vi "mainlockin2.vi"() -> ()   [LabVIEW 2021]
panel:
  out "outputdc 2":dbl[](array[numeric]) format="%.2f"
  in  "GPIB address dc meter 2":string
  out "dup directory path":path
  in  "GPIB address dc meter":string
  in  "GPIB  address  lockin":string
  in  "GPIB address magnet":string
  in  "GPIB address Temp controller":string
  in  "Wait (minute)":sgl
  in  "No of Temp Steps":i16
  in  "folder name to save files":string
  out "outputtemp":dbl[](array[numeric]) format="%.2f"
  out "outputdc":dbl[](array[numeric]) format="%.2f"
  out "outputlockin 2":dbl[](array[numeric]) format="%.2f"
  out "outputlockin 1":dbl[](array[numeric]) format="%.2f"
  out "field":dbl[](array[numeric]) format="%.2f"
  out "Current Temp":dbl format="%.3f"
  in  "Increasing \nTemp step":bool=TRUE
  in  "Temperature\nInterval":dbl format="%.3f"
  in  "Initial Temp C":dbl format="%.3f"
  # "Help:\n1. write the folder name to save the files.The file name will \nbe the temperature in the given folder.\n2.Write the GPIB address of all the instruments before running\nthe program.\n3. Give the initial temperature and the temperature interval \nand the total number of steps.\n4.Check whether you want to increase the temperature or\ndecrease.\n5.Write the time to be waited to let the tempetature controller\nequilibrate.\n6.Once the speps 1 through 5 is done run the experiment."
  # "Decreasing\nTemp Step"
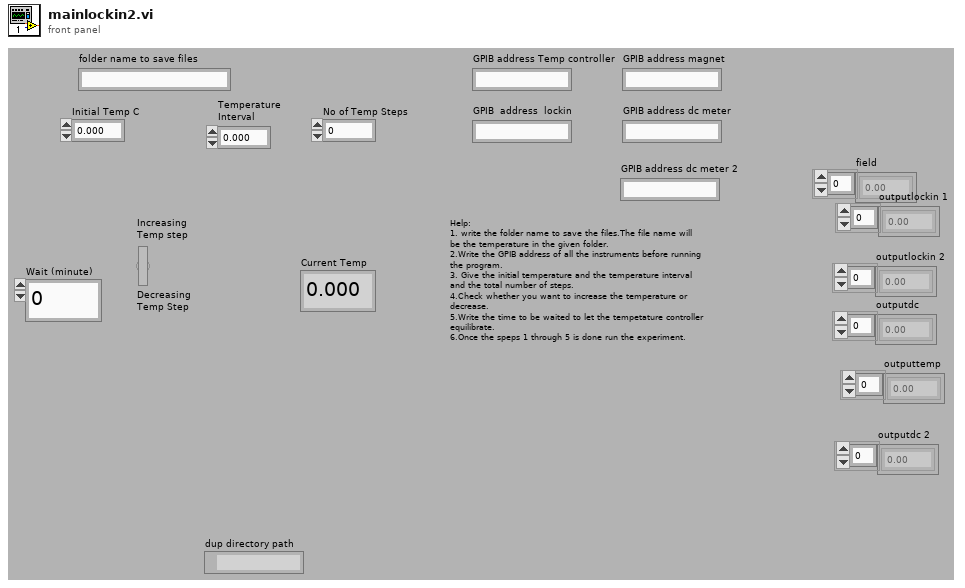
[diagram p1: front panel]
types:
  T1 = enum16{"--Quit--", "Read-Status", "Read-Cell", "Read-Field[T]", "Read-Setpoint[T]"}
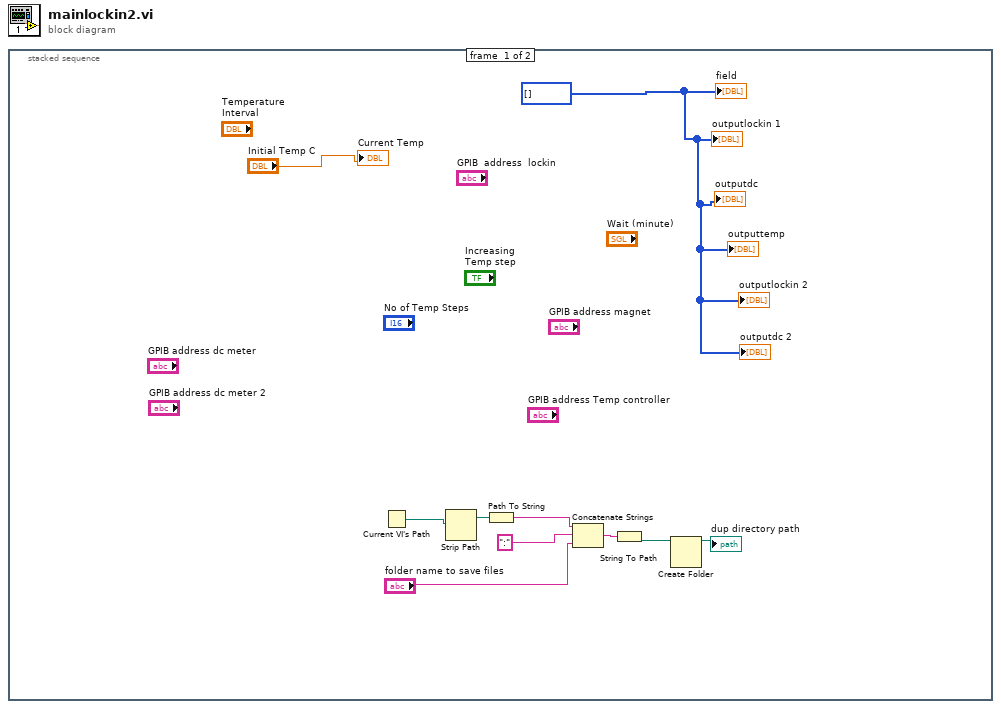
[diagram p0: block diagram]
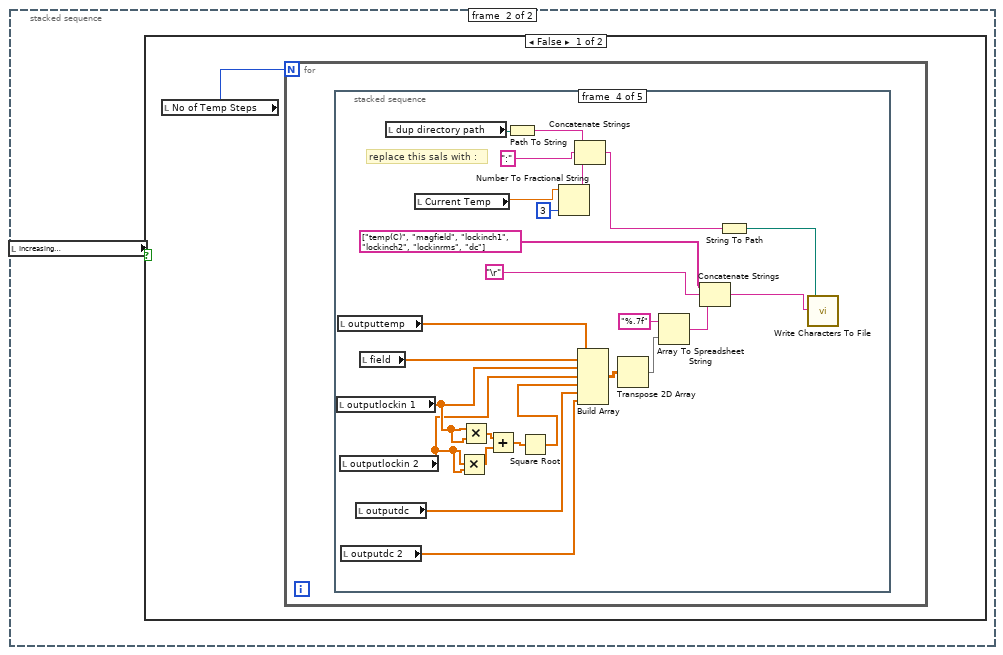
[diagram p2: hidden frame]
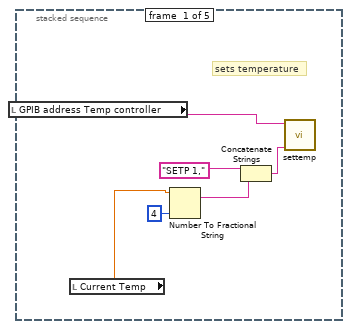
[diagram p3: hidden frame]
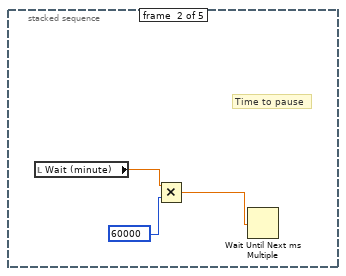
[diagram p4: hidden frame]
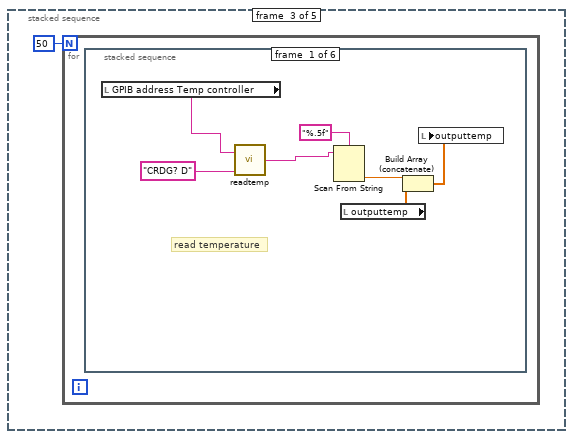
[diagram p5: hidden frame]
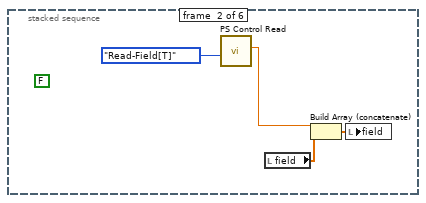
[diagram p6: hidden frame]
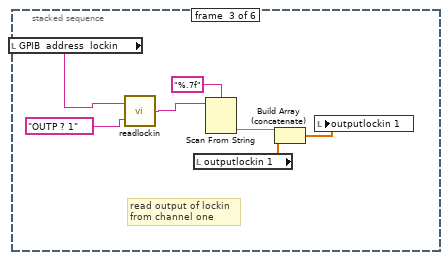
[diagram p7: hidden frame]
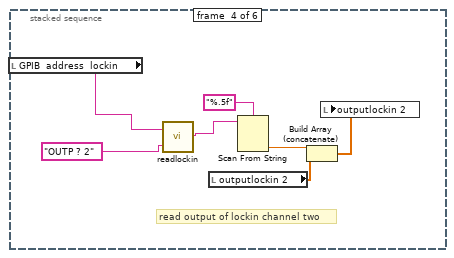
[diagram p8: hidden frame]
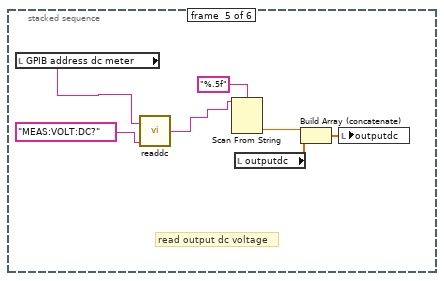
[diagram p9: hidden frame]
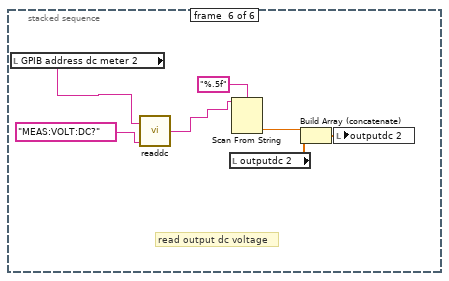
[diagram p10: hidden frame]
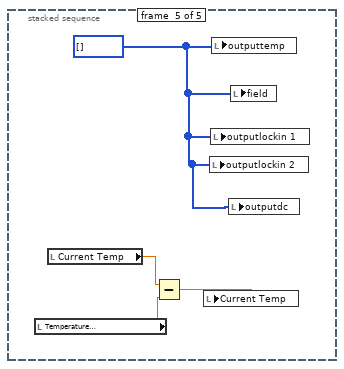
[diagram p11: hidden frame]
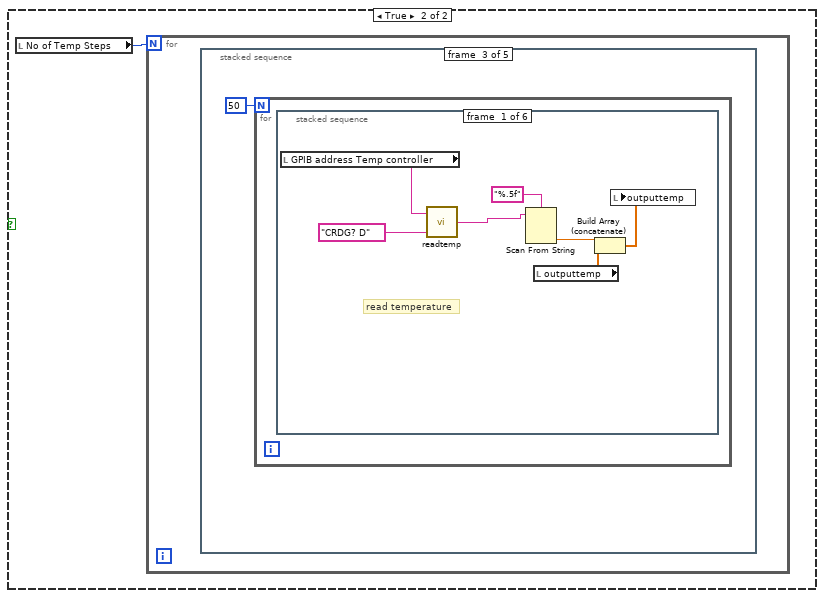
[diagram p12: hidden frame]
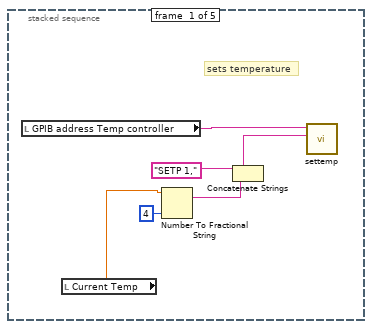
[diagram p13: hidden frame]
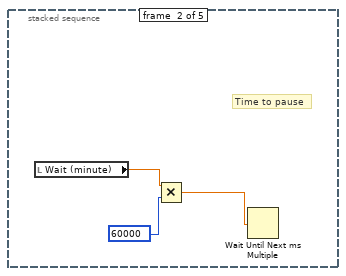
[diagram p14: hidden frame]
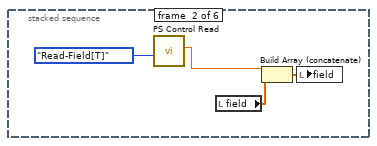
[diagram p15: hidden frame]
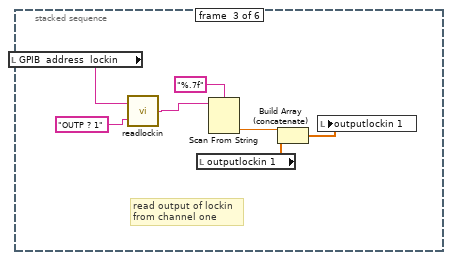
[diagram p16: hidden frame]
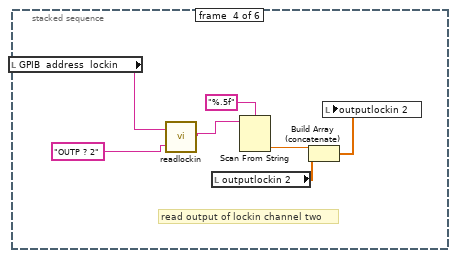
[diagram p17: hidden frame]
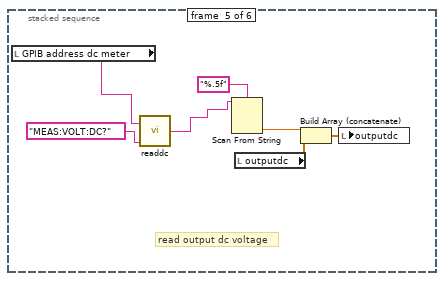
[diagram p18: hidden frame]
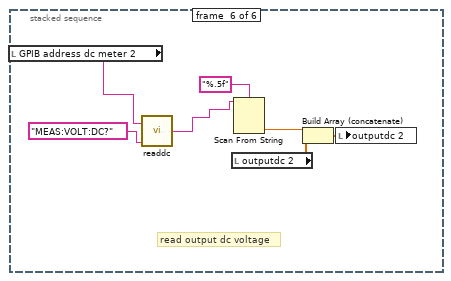
[diagram p19: hidden frame]
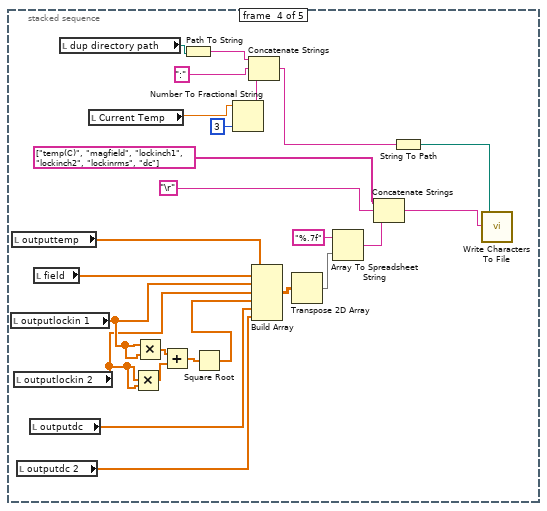
[diagram p20: hidden frame]
diagram:
  n1 = stacked-sequence {
    frame #0 {
      w1 = i32[] [] ("field")
      n2 = Current VI's Path() -> (path=w9:path)
      n3 = Strip Path(path=w9) -> (stripped path=w8:path)  [unwired: 1 out]
      n4 = Path To String(path=w8) -> (string=w7:string)
      n5 = Concatenate Strings(w7, ":", "folder name to save files") -> (w4:string)
      n6 = String To Path(string=w4) -> (path=w3:path)
      n7 = Create Folder(path (use dialog)=w3) -> (created path=→"dup directory path":path)  [unwired: 2 in, 2 out]
      "Current Temp" <- "Initial Temp C"
      "field" <- w1
      "outputlockin 1" <- w1
      "outputdc" <- w1
      "outputtemp" <- w1
      "outputlockin 2" <- w1
      "outputdc 2" <- w1
    }
    frame #1 {
      n8 = local read "Increasing \nTemp step"() -> (w11:bool)
      n9 = case shown="False" w11 {
        frame False {
          n10 = local read "No of Temp Steps"() -> (w12:i16)
          n11 = for {
            N: w12 -> [_]
            n12 = stacked-sequence {
              frame #0 {
                # "sets temperature"
                n13 = local read "GPIB address Temp controller"() -> (w13:string)
                n14 = local read "Current Temp"() -> (w15:dbl)
                n15 = Number To Fractional String(number=w15, precision (6)=i16 4) -> (F-format string=w18:string)  [unwired: 2 in]
                n16 = Concatenate Strings("SETP 1,", w18) -> (w16:string)
                n17 = call "settemp.vi"("Characters to Write"=w16, "GPIB\nAddress"=w13) -> ()  [unwired: 5 in, 1 out]
              }
              frame #1 {
                # "Time to pause"
                n18 = local read "Wait (minute)"() -> (w21:sgl)
                n19 = Multiply(x=w21, y=u32 60000 ("millisecond multiple")) -> (x*y=w19:sgl)
                n20 = Wait Until Next ms Multiple(millisecond multiple=w19) -> ()  [unwired: 1 out]
              }
              frame #2 {
                n21 = for {
                  N: 50 -> [_]
                  n22 = stacked-sequence {
                    frame #0 {
                      # "read temperature"
                      n23 = local read "GPIB address Temp controller"() -> (w23:string)
                      n24 = call "readtemp.vi"("Characters to Write"="CRDG? D", "GPIB\nAddress"=w23) -> ("Characters Read"=w24:string)
                      n25 = Scan From String(format string="%.5f", input string=w24) -> (output 1=w26:dbl)  [unwired: 3 in, 3 out]
                      n26 = local read "outputtemp"() -> (w29:dbl[])
                      n27 = Build Array (concatenate)(w26, w29) -> (w28:dbl[])
                      n28 = local write "outputtemp"(w28) -> ()
                    }
                    frame #1 {
                      (unwired) FALSE
                      n29 = call "PS Control Read.vi"("Read State"=T1."Read-Field[T]") -> ("Current Field"=w30:dbl)  [unwired: 3 in, 4 out]
                      n30 = local read "field"() -> (w32:dbl[])
                      n31 = Build Array (concatenate)(w30, w32) -> (w31:dbl[])
                      n32 = local write "field"(w31) -> ()
                    }
                    frame #2 {
                      # "read output of lockin\nfrom channel one"
                      n33 = local read "GPIB  address  lockin"() -> (w34:string)
                      n34 = call "readlockin.vi"("Characters to Write"="OUTP ? 1", "GPIB\nAddress"=w34) -> ("Characters Read"=w35:string)
                      n35 = local read "outputlockin 1"() -> (w39:dbl[])
                      n36 = Scan From String(format string="%.7f", input string=w35) -> (output 1=w36:dbl)  [unwired: 3 in, 3 out]
                      n37 = Build Array (concatenate)(w36, w39) -> (w38:dbl[])
                      n38 = local write "outputlockin 1"(w38) -> ()
                    }
                    frame #3 {
                      # "read output of lockin channel two"
                      n39 = local read "GPIB  address  lockin"() -> (w41:string)
                      n40 = call "readlockin.vi"("Characters to Write"="OUTP ? 2", "GPIB\nAddress"=w41) -> ("Characters Read"=w42:string)
                      n41 = local read "outputlockin 2"() -> (w46:dbl[])
                      n42 = Scan From String(format string="%.5f", input string=w42) -> (output 1=w44:dbl)  [unwired: 3 in, 3 out]
                      n43 = Build Array (concatenate)(w44, w46) -> (w45:dbl[])
                      n44 = local write "outputlockin 2"(w45) -> ()
                    }
                    frame #4 {
                      # "read output dc voltage"
                      n45 = local read "GPIB address dc meter"() -> (w48:string)
                      n46 = call "readdc.vi"("Characters to Write"="MEAS:VOLT:DC?", "GPIB\nAddress"=w48) -> ("Characters Read"=w49:string)
                      n47 = Scan From String(format string="%.5f", input string=w49) -> (output 1=w51:dbl)  [unwired: 3 in, 3 out]
                      n48 = local read "outputdc"() -> (w54:dbl[])
                      n49 = Build Array (concatenate)(w51, w54) -> (w53:dbl[])
                      n50 = local write "outputdc"(w53) -> ()
                    }
                    frame #5 {
                      # "read output dc voltage"
                      n51 = local read "GPIB address dc meter 2"() -> (w55:string)
                      n52 = call "readdc.vi"("Characters to Write"="MEAS:VOLT:DC?", "GPIB\nAddress"=w55) -> ("Characters Read"=w56:string)
                      n53 = local read "outputdc 2"() -> (w61:dbl[])
                      n54 = Scan From String(format string="%.5f", input string=w56) -> (output 1=w58:dbl)  [unwired: 3 in, 3 out]
                      n55 = Build Array (concatenate)(w58, w61) -> (w60:dbl[])
                      n56 = local write "outputdc 2"(w60) -> ()
                    }
                  }
                }
              }
              frame #3 {
                # "replace this sals with :"
                n57 = local read "outputlockin 1"() -> (w79:dbl[])
                n58 = local read "outputtemp"() -> (w81:dbl[])
                n59 = local read "outputlockin 2"() -> (w78:dbl[])
                n60 = local read "outputdc 2"() -> (w62:dbl[])
                n61 = local read "outputdc"() -> (w73:dbl[])
                n62 = local read "field"() -> (w80:dbl[])
                n63 = local read "dup directory path"() -> (w64:path)
                n64 = local read "Current Temp"() -> (w83:dbl)
                n65 = Multiply(x=w78, y=w78) -> (x*y=w76:dbl[])
                n66 = Multiply(x=w79, y=w79) -> (x*y=w77:dbl[])
                n67 = Add(x=w77, y=w76) -> (x+y=w75:dbl[])
                n68 = Path To String(path=w64) -> (string=w63:string)
                n69 = Square Root(x=w75) -> (sqrt(x)=w74:dbl[])
                n70 = Number To Fractional String(number=w83, precision (6)=i16 3) -> (F-format string=w82:string)  [unwired: 2 in]
                n71 = Concatenate Strings(w63, ":", w82) -> (w85:string)
                n72 = Build Array(w81, w80, w79, w78, w74, w73, w62) -> (w72:dbl[][])
                n73 = Transpose 2D Array(2D array=w72) -> (transposed array=w70:dbl[][])
                n74 = Array To Spreadsheet String(array=w70, 3:"%.7f" ("format string")) -> (spreadsheet string=w67:string)  [unwired: 1 in]
                n75 = Concatenate Strings(string[] ["temp(C)", "magfield", "lockinch1", "lockinch2", "lockinrms", "dc"], "\r", w67) -> (w66:string)
                n76 = String To Path(string=w85) -> (path=w84:path)
                n77 = call <vilib>:"Write Characters To File.vi"("character string"=w66, "file path (dialog if empty)"=w84) -> ()  [unwired: 3 in, 1 out]
              }
              frame #4 {
                w90 = i32[] []
                n78 = local read "Temperature\nInterval"() -> (w88:dbl)
                n79 = local read "Current Temp"() -> (w89:dbl)
                n80 = Subtract(x=w89, y=w88) -> (x-y=w87:dbl)
                n81 = local write "Current Temp"(w87) -> ()
                n82 = local write "outputlockin 2"(w90) -> ()
                n83 = local write "outputlockin 1"(w90) -> ()
                n84 = local write "outputtemp"(w90) -> ()
                n85 = local write "outputdc"(w90) -> ()
                n86 = local write "field"(w90) -> ()
              }
            }
          }
        }
        frame True {
          n87 = local read "No of Temp Steps"() -> (w91:i16)
          n88 = for {
            N: w91 -> [_]
            n89 = stacked-sequence {
              frame #0 {
                # "sets temperature"
                n90 = local read "GPIB address Temp controller"() -> (w92:string)
                n91 = local read "Current Temp"() -> (w94:dbl)
                n92 = Number To Fractional String(number=w94, precision (6)=i16 4) -> (F-format string=w97:string)  [unwired: 2 in]
                n93 = Concatenate Strings("SETP 1,", w97) -> (w95:string)
                n94 = call "settemp.vi"("Characters to Write"=w95, "GPIB\nAddress"=w92) -> ()  [unwired: 5 in, 1 out]
              }
              frame #1 {
                # "Time to pause"
                n95 = local read "Wait (minute)"() -> (w100:sgl)
                n96 = Multiply(x=w100, y=u32 60000 ("millisecond multiple")) -> (x*y=w98:sgl)
                n97 = Wait Until Next ms Multiple(millisecond multiple=w98) -> ()  [unwired: 1 out]
              }
              frame #2 {
                n98 = for {
                  N: 50 -> [_]
                  n99 = stacked-sequence {
                    frame #0 {
                      # "read temperature"
                      n100 = local read "GPIB address Temp controller"() -> (w102:string)
                      n101 = call "readtemp.vi"("Characters to Write"="CRDG? D", "GPIB\nAddress"=w102) -> ("Characters Read"=w103:string)
                      n102 = Scan From String(format string="%.5f", input string=w103) -> (output 1=w105:dbl)  [unwired: 3 in, 3 out]
                      n103 = local read "outputtemp"() -> (w108:dbl[])
                      n104 = Build Array (concatenate)(w105, w108) -> (w107:dbl[])
                      n105 = local write "outputtemp"(w107) -> ()
                    }
                    frame #1 {
                      n106 = call "PS Control Read.vi"("Read State"=T1."Read-Field[T]") -> ("Current Field"=w109:dbl)  [unwired: 3 in, 4 out]
                      n107 = local read "field"() -> (w111:dbl[])
                      n108 = Build Array (concatenate)(w109, w111) -> (w110:dbl[])
                      n109 = local write "field"(w110) -> ()
                    }
                    frame #2 {
                      # "read output of lockin\nfrom channel one"
                      n110 = local read "GPIB  address  lockin"() -> (w113:string)
                      n111 = call "readlockin.vi"("Characters to Write"="OUTP ? 1", "GPIB\nAddress"=w113) -> ("Characters Read"=w114:string)
                      n112 = local read "outputlockin 1"() -> (w118:dbl[])
                      n113 = Scan From String(format string="%.7f", input string=w114) -> (output 1=w115:dbl)  [unwired: 3 in, 3 out]
                      n114 = Build Array (concatenate)(w115, w118) -> (w117:dbl[])
                      n115 = local write "outputlockin 1"(w117) -> ()
                    }
                    frame #3 {
                      # "read output of lockin channel two"
                      n116 = local read "GPIB  address  lockin"() -> (w120:string)
                      n117 = call "readlockin.vi"("Characters to Write"="OUTP ? 2", "GPIB\nAddress"=w120) -> ("Characters Read"=w121:string)
                      n118 = local read "outputlockin 2"() -> (w125:dbl[])
                      n119 = Scan From String(format string="%.5f", input string=w121) -> (output 1=w123:dbl)  [unwired: 3 in, 3 out]
                      n120 = Build Array (concatenate)(w123, w125) -> (w124:dbl[])
                      n121 = local write "outputlockin 2"(w124) -> ()
                    }
                    frame #4 {
                      # "read output dc voltage"
                      n122 = local read "GPIB address dc meter"() -> (w127:string)
                      n123 = call "readdc.vi"("Characters to Write"="MEAS:VOLT:DC?", "GPIB\nAddress"=w127) -> ("Characters Read"=w128:string)
                      n124 = Scan From String(format string="%.5f", input string=w128) -> (output 1=w130:dbl)  [unwired: 3 in, 3 out]
                      n125 = local read "outputdc"() -> (w133:dbl[])
                      n126 = Build Array (concatenate)(w130, w133) -> (w132:dbl[])
                      n127 = local write "outputdc"(w132) -> ()
                    }
                    frame #5 {
                      # "read output dc voltage"
                      n128 = local read "GPIB address dc meter 2"() -> (w134:string)
                      n129 = call "readdc.vi"("Characters to Write"="MEAS:VOLT:DC?", "GPIB\nAddress"=w134) -> ("Characters Read"=w135:string)
                      n130 = local read "outputdc 2"() -> (w140:dbl[])
                      n131 = Scan From String(format string="%.5f", input string=w135) -> (output 1=w137:dbl)  [unwired: 3 in, 3 out]
                      n132 = Build Array (concatenate)(w137, w140) -> (w139:dbl[])
                      n133 = local write "outputdc 2"(w139) -> ()
                    }
                  }
                }
              }
              frame #3 {
                n134 = local read "outputlockin 1"() -> (w158:dbl[])
                n135 = local read "outputtemp"() -> (w160:dbl[])
                n136 = local read "outputlockin 2"() -> (w157:dbl[])
                n137 = local read "outputdc 2"() -> (w141:dbl[])
                n138 = local read "outputdc"() -> (w152:dbl[])
                n139 = local read "field"() -> (w159:dbl[])
                n140 = local read "dup directory path"() -> (w143:path)
                n141 = local read "Current Temp"() -> (w162:dbl)
                n142 = Multiply(x=w157, y=w157) -> (x*y=w155:dbl[])
                n143 = Multiply(x=w158, y=w158) -> (x*y=w156:dbl[])
                n144 = Add(x=w156, y=w155) -> (x+y=w154:dbl[])
                n145 = Path To String(path=w143) -> (string=w142:string)
                n146 = Square Root(x=w154) -> (sqrt(x)=w153:dbl[])
                n147 = Number To Fractional String(number=w162, precision (6)=i16 3) -> (F-format string=w161:string)  [unwired: 2 in]
                n148 = Concatenate Strings(w142, ":", w161) -> (w164:string)
                n149 = Build Array(w160, w159, w158, w157, w153, w152, w141) -> (w151:dbl[][])
                n150 = Transpose 2D Array(2D array=w151) -> (transposed array=w149:dbl[][])
                n151 = Array To Spreadsheet String(array=w149, 3:"%.7f" ("format string")) -> (spreadsheet string=w146:string)  [unwired: 1 in]
                n152 = Concatenate Strings(string[] ["temp(C)", "magfield", "lockinch1", "lockinch2", "lockinrms", "dc"], "\r", w146) -> (w145:string)
                n153 = String To Path(string=w164) -> (path=w163:path)
                n154 = call <vilib>:"Write Characters To File.vi"("character string"=w145, "file path (dialog if empty)"=w163) -> ()  [unwired: 3 in, 1 out]
              }
              frame #4 {
                w169 = i32[] []
                n155 = local read "Temperature\nInterval"() -> (w167:dbl)
                n156 = local read "Current Temp"() -> (w168:dbl)
                n157 = Add(x=w168, y=w167) -> (x+y=w166:dbl)
                n158 = local write "Current Temp"(w166) -> ()
                n159 = local write "outputlockin 2"(w169) -> ()
                n160 = local write "outputlockin 1"(w169) -> ()
                n161 = local write "outputtemp"(w169) -> ()
                n162 = local write "outputdc"(w169) -> ()
                n163 = local write "field"(w169) -> ()
              }
            }
          }
        }
      }
    }
  }
